vi "Measure Suply IV.vi"(0 "Supply Line Handle in":refnum<k15>, 11 "error in (no error)":errorcluster) -> (4 "Supply Line Handle out":refnum<k15>, 6 "Current Measurement":dbl, 8 "Voltage Measurement":dbl, 15 "error out":errorcluster)   [LabVIEW 2018, in "SMU.lvlib"]
uses:
  SMU.lvlib
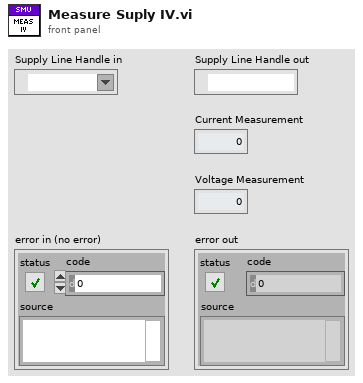
[diagram p1: front panel]
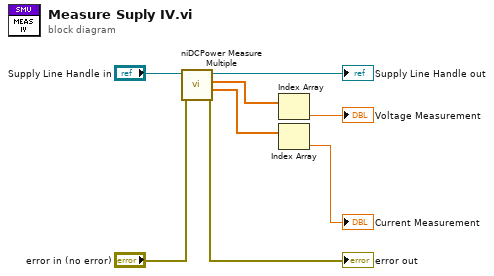
[diagram p0: block diagram]
diagram:
  n1 = call <instrlib>:"niDCPower Measure Multiple.vi"("error in (no error)"="error in (no error)", "instrument handle"="Supply Line Handle in") -> ("error out"=→"error out":errorcluster, "current measurements"=w5:dbl[], "voltage measurements"=w6:dbl[], "instrument handle out"=→"Supply Line Handle out":refnum<k15>)  [unwired: 6 in]
  n2 = Index Array(array=w6) -> (element=→"Voltage Measurement":dbl)  [unwired: 1 in]
  n3 = Index Array(array=w5) -> (element=→"Current Measurement":dbl)  [unwired: 1 in]
